vi "Correct LCOS Pattern.vi"(0 "Images Dest":T1, 1 "Pattern":enum16{"Computed", "From File", "Correction"}(ring), 3 "error in":errorcluster) -> (6 "Images Out":T1, 9 "error out":errorcluster)   [LabVIEW 2011]
uses:
  LCOS Images.ctl
  <vilib>/vision/Image Controls.llb/IMAQ Image.ctl
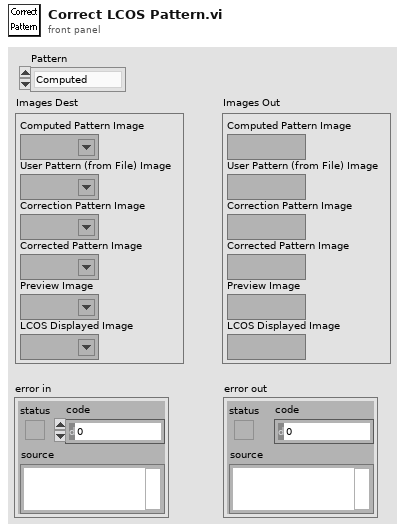
[diagram p1: front panel]
types:
  T1 = typedef "LCOS Images.ctl" = cluster{"Computed Pattern Image":T2, "User Pattern (from File) Image":T2, "Correction Pattern Image":T2, "Corrected Pattern Image":T2, "Preview Image":T2, "LCOS Displayed Image":T2}
  T2 = typedef "IMAQ Image.ctl" = refnum<image>
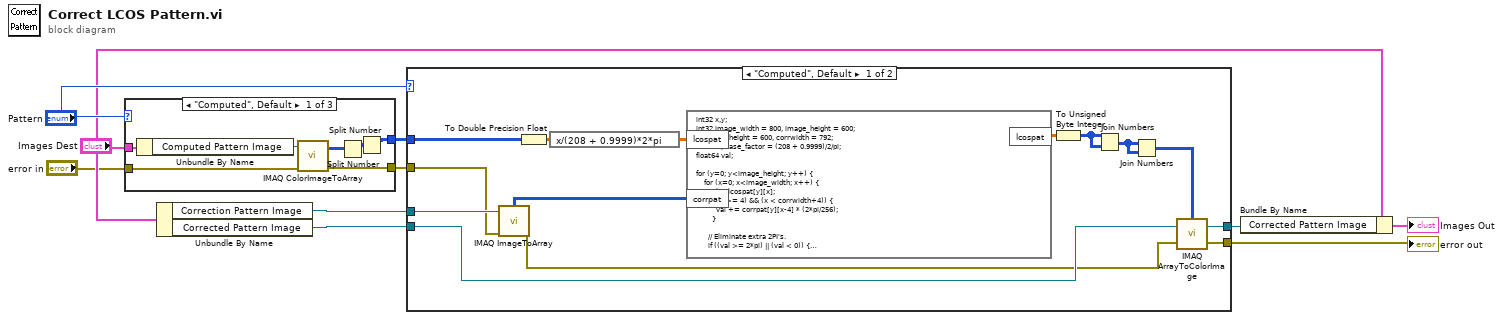
[diagram p0: block diagram]
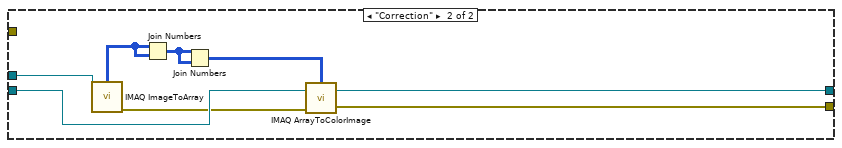
[diagram p2: hidden frame]
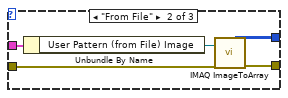
[diagram p3: hidden frame]
diagram:
  n1 = case shown="\"Computed\", Default" "Pattern" {
    tunnel: "Images Dest" -> [w17 w22 _]
    tunnel: "error in" -> [w15 w20 w23]
    tunnel: [w12 w19 _] -> w2
    tunnel: [w11 w18 w23] -> w1
    frame "Computed", Default {
      n2 = Unbundle By Name(w17) -> ("Computed Pattern Image"=w16:T2)
      n3 = call "IMAQ ColorImageToArray"("Image"=w16, "error in (no error)"=w15) -> ("Image Pixels (U32)"=w13:u32[][], "error out"=w11:errorcluster)  [unwired: 2 in, 1 out]
      n4 = Split Number(x=w13) -> (hi(x)=w14:u16[][])  [unwired: 1 out]
      n5 = Split Number(x=w14) -> (hi(x)=w12:u8[][])  [unwired: 1 out]
    }
    frame "From File" {
      n6 = Unbundle By Name(w22) -> ("User Pattern (from File) Image"=w21:T2)
      n7 = call "IMAQ ImageToArray"("error in (no error)"=w20, "Image"=w21) -> ("error out"=w18:errorcluster, "Image Pixels (U8)"=w19:u8[][])  [unwired: 2 in, 3 out]
    }
    frame "Correction" {
    }
  }
  n8 = Unbundle By Name("Images Dest") -> ("Correction Pattern Image"=w9:T2, "Corrected Pattern Image"=w5:T2)
  n9 = case shown="\"Computed\", Default" "Pattern" {
    tunnel: w9 -> [w37 w45]
    tunnel: [w31 w39] -> w7
    tunnel: w5 -> [w30 w41]
    tunnel: [w28 w38] -> w4
    tunnel: w2 -> [w25 _]
    tunnel: w1 -> [w24 _]
    frame "Computed", Default {
      n10 = call "IMAQ ImageToArray"("error in (no error)"=w24, "Image"=w37) -> ("error out"=w29:errorcluster, "Image Pixels (U8)"=w27:u8[][])  [unwired: 2 in, 3 out]
      n11 = To Double Precision Float(number=w25) -> (double precision float=w26:dbl[][])
      n12 = expression code="x/(208 + 0.9999)*2*pi"(w26) -> (w36:dbl[][])
      n13 = formula code="int32 x,y;\nint32 image_width = 800, image_height = 600;\nint32 corrheight = 600, corrwidth = 792;\nfloat64 phase_factor = (208 + 0.9999)/2/pi;\nfloat64 val;\n\nfor (y=0; y<image_height; y++) {\n    for (x=0; x<image_width; x++) {\n      val = lcospat[y][x];\n      if ((x >= 4) && (x < corrwidth+4)) {\n          val += corrpat[y][x-4] * (2*pi/256);\n        }\n\n      // Eliminate extra 2PI's.\n      if ((val >= 2*pi) || (val < 0)) {\n        val = val-floor(val/2/pi)*2*pi;\n      }\t\n\n      // Map 2PI to correct greyscale value.\n      val = val * phase_factor;\n\n      lcospat[y][x] = val;\n  }\n}"("lcospat"=w36, "corrpat"=w27) -> ("lcospat"=w35:dbl[][])
      n14 = To Unsigned Byte Integer(number=w35) -> (unsigned 8bit integer=w34:u8[][])
      n15 = Join Numbers(hi=w34, lo=w34) -> ((hi.lo)=w33:u16[][])
      n16 = Join Numbers(hi=w33, lo=w33) -> ((hi.lo)=w32:u32[][])
      n17 = call "IMAQ ArrayToColorImage"("Image Pixels (U32)"=w32, "Image"=w30, "error in (no error)"=w29) -> ("Image Out"=w31:T2, "error out"=w28:errorcluster)  [unwired: 2 in]
    }
    frame "Correction" {
      n18 = call "IMAQ ImageToArray"("Image"=w45) -> ("error out"=w40:errorcluster, "Image Pixels (U8)"=w44:u8[][])  [unwired: 3 in, 3 out]
      n19 = Join Numbers(hi=w44, lo=w44) -> ((hi.lo)=w43:u16[][])
      n20 = Join Numbers(hi=w43, lo=w43) -> ((hi.lo)=w42:u32[][])
      n21 = call "IMAQ ArrayToColorImage"("Image Pixels (U32)"=w42, "Image"=w41, "error in (no error)"=w40) -> ("Image Out"=w39:T2, "error out"=w38:errorcluster)  [unwired: 2 in]
    }
  }
  "error out" <- w4
  n22 = Bundle By Name(cluster="Images Dest", "Corrected Pattern Image"=w7) -> (→"Images Out":T1)
